vi "Day 1 Puzzle 2.vi"() -> ()   [LabVIEW 2021]
panel:
  out "result":i64
  out "max value 3":i64
  out "max value 2":i64
  out "max value 1":i64
  in  "Path":path
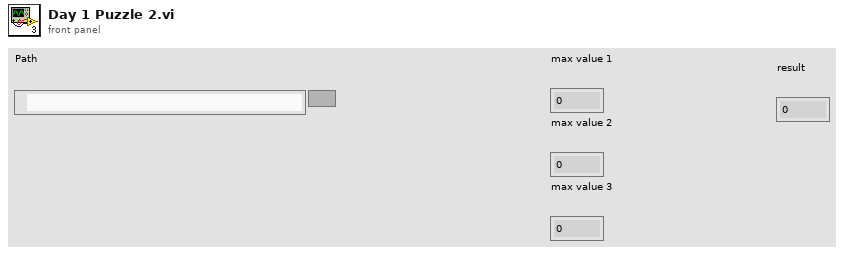
[diagram p1: front panel]
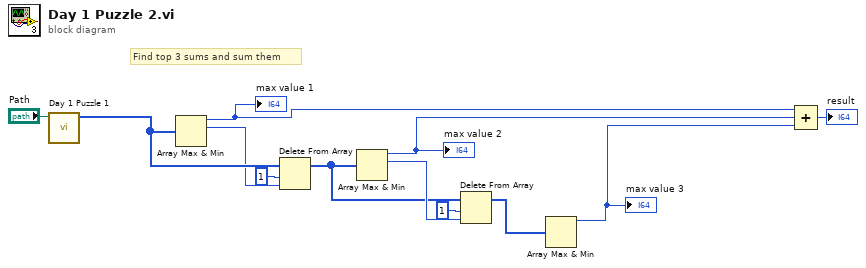
[diagram p0: block diagram]
diagram:
  # "Find top 3 sums and sum them"
  n1 = call "Day 1 Puzzle 1.vi"("Path"="Path") -> ("Snacks sum list"=w11:i64[])  [unwired: 10 in]
  n2 = Array Max & Min(array=w11) -> (max value=w4:i64, max index (indices)=w9:i32)  [unwired: 2 out]
  "max value 1" <- w4
  n3 = Delete From Array(array=w11, length=1, index=w9) -> (array with subset deleted=w6:i64[])  [unwired: 1 out]
  n4 = Array Max & Min(array=w6) -> (max value=w3:i64, max index (indices)=w7:i32)  [unwired: 2 out]
  "max value 2" <- w3
  n5 = Delete From Array(array=w6, length=1, index=w7) -> (array with subset deleted=w5:i64[])  [unwired: 1 out]
  n6 = Array Max & Min(array=w5) -> (max value=w2:i64)  [unwired: 3 out]
  "max value 3" <- w2
  n7 = Compound Arithmetic op=ADD(w4, w3, w2) -> (→"result":i64)
